vi "CG test stand DAQ main.vi"() -> ()   [LabVIEW 2020]
doc: "This example demonstrates how to read N channels of analog input from a LINX device."
uses:
  <vilib>/MakerHub/LINX/Public/Peripherals/Analog/Analog Read N Chans.vi
  <vilib>/MakerHub/LINX/Private/Local IO/LinxAnalogRead.vi
  <vilib>/MakerHub/LINX/Public/Utilities/Check Channel.vi
  <vilib>/MakerHub/LINX/Public/Utilities/Open Serial.vi
  <vilib>/MakerHub/LINX/Private/Utilties/Generate Error.vi
  <vilib>/Analysis/Matrix/Numeric/Conversions/Array To Matrix - RA.vi
  <vilib>/Utility/file.llb/Write Delimited Spreadsheet (DBL).vi
  <vilib>/MakerHub/LINX/LMH-LINX.lvlib
  <vilib>/Analysis/Matrix/NI_Matrix.lvlib
panel:
  out "Temperatures":dbl[](graph)
  out "Pressures":dbl[](graph)
  out "TC3 (KOhm)":dbl
  out "TC2 (KOhm)":dbl
  out "TC1 (KOhm)":dbl
  out "Throat Pressure (PSI)":dbl
  out "Inlet Pressure (PSI)":dbl
  out "Throat temperature (K)":dbl(slide) scale=0.0..250.0
  out "Inlet temperature (K)":dbl(slide) scale=0.0..250.0
  out "Tank temperature (K)":dbl(slide) scale=0.0..250.0
  out "Throat Pressure (PSI)":dbl(knob) scale=0.0..100.0
  out "Inlet Pressure (PSI)":dbl(knob) scale=0.0..100.0
  out "WRITING TO FILE":bool
  in  "?":bool
  out "error out":errorcluster
  out "Full filepath":string
  in  "Path":path
  in  "File extension":string
  in  "Filename":string
  in  "Wait time (ms)":dbl
  out "Time":timestamp
  in  "Stop Button":bool
  out "Loop Rate (Hz)":u32
  in  "Serial Port":refnum<visa-resource-name>
  # "File I/O"
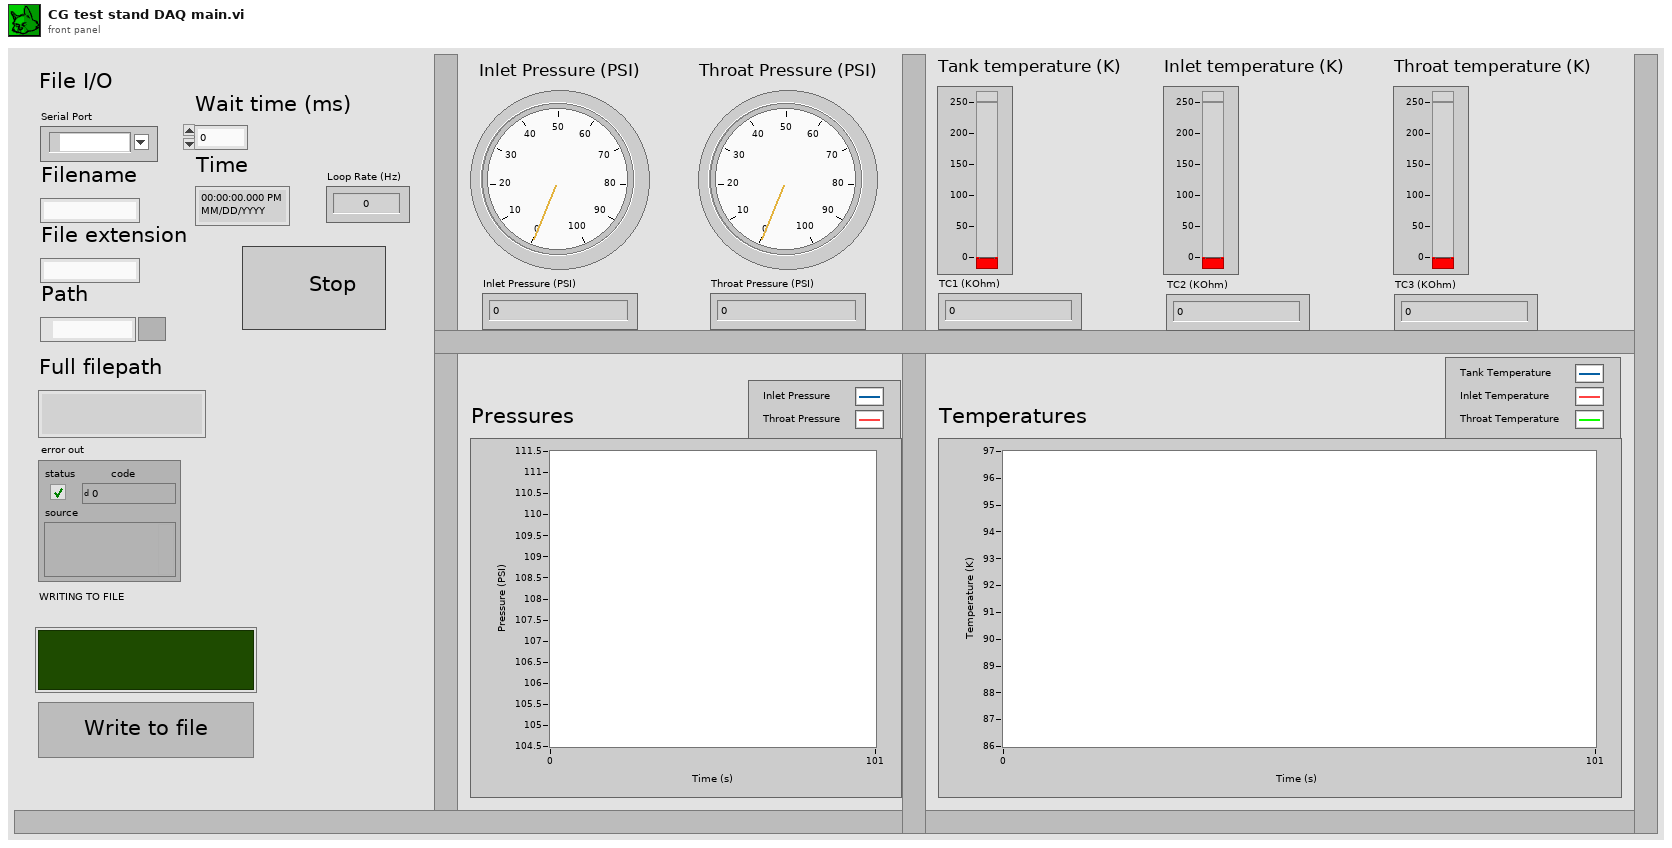
[diagram p1: front panel]
types:
  T1 = typedef "LMH-LINX.lvlib/LINX Ref.ctl" = cluster{"IO":T2, "Interface":T3, "LINX Device Config":T4}
  T2 = typedef "LMH-LINX.lvlib/Platform.ctl" = enum16{"Remote", "Local"}
  T3 = typedef "LMH-LINX.lvlib/Interface.ctl" = enum16{"Serial", "TCP"}
  T4 = typedef "LMH-LINX.lvlib/Device.lvlib/LINX Device Config.ctl" = cluster{"Interface":T3, "COM Port":refnum<visa-resource-name>, "TCP Configuration":T5, "Device Family":u8, "Device ID":u8, "Device Name":string, "TCP Ref":refnum<k5>, "Channels":T6}
  T5 = typedef "LMH-LINX.lvlib/Device.lvlib/TCP Config.ctl" = cluster{"IP Address":string, "Port":u16}
  T6 = typedef "LMH-LINX.lvlib/Channels.ctl" = cluster{"DI":u8[], "DO":u8[], "AI":u8[], "AO":u8[], "PWM":u8[], "QE":u8[], "UART":u8[], "I2C 2":u8[], "SPI":u8[], "CAN":u8[], "Servo":u8[], "AI Ref (V)":dbl, "AI Resolution (Bits)":u8, "AO Ref (V)":dbl, "AO Resolution (Bits)":u8}
  T7 = typedef "NI_Matrix.lvlib/RealMatrix.ctl" = dbl[][]
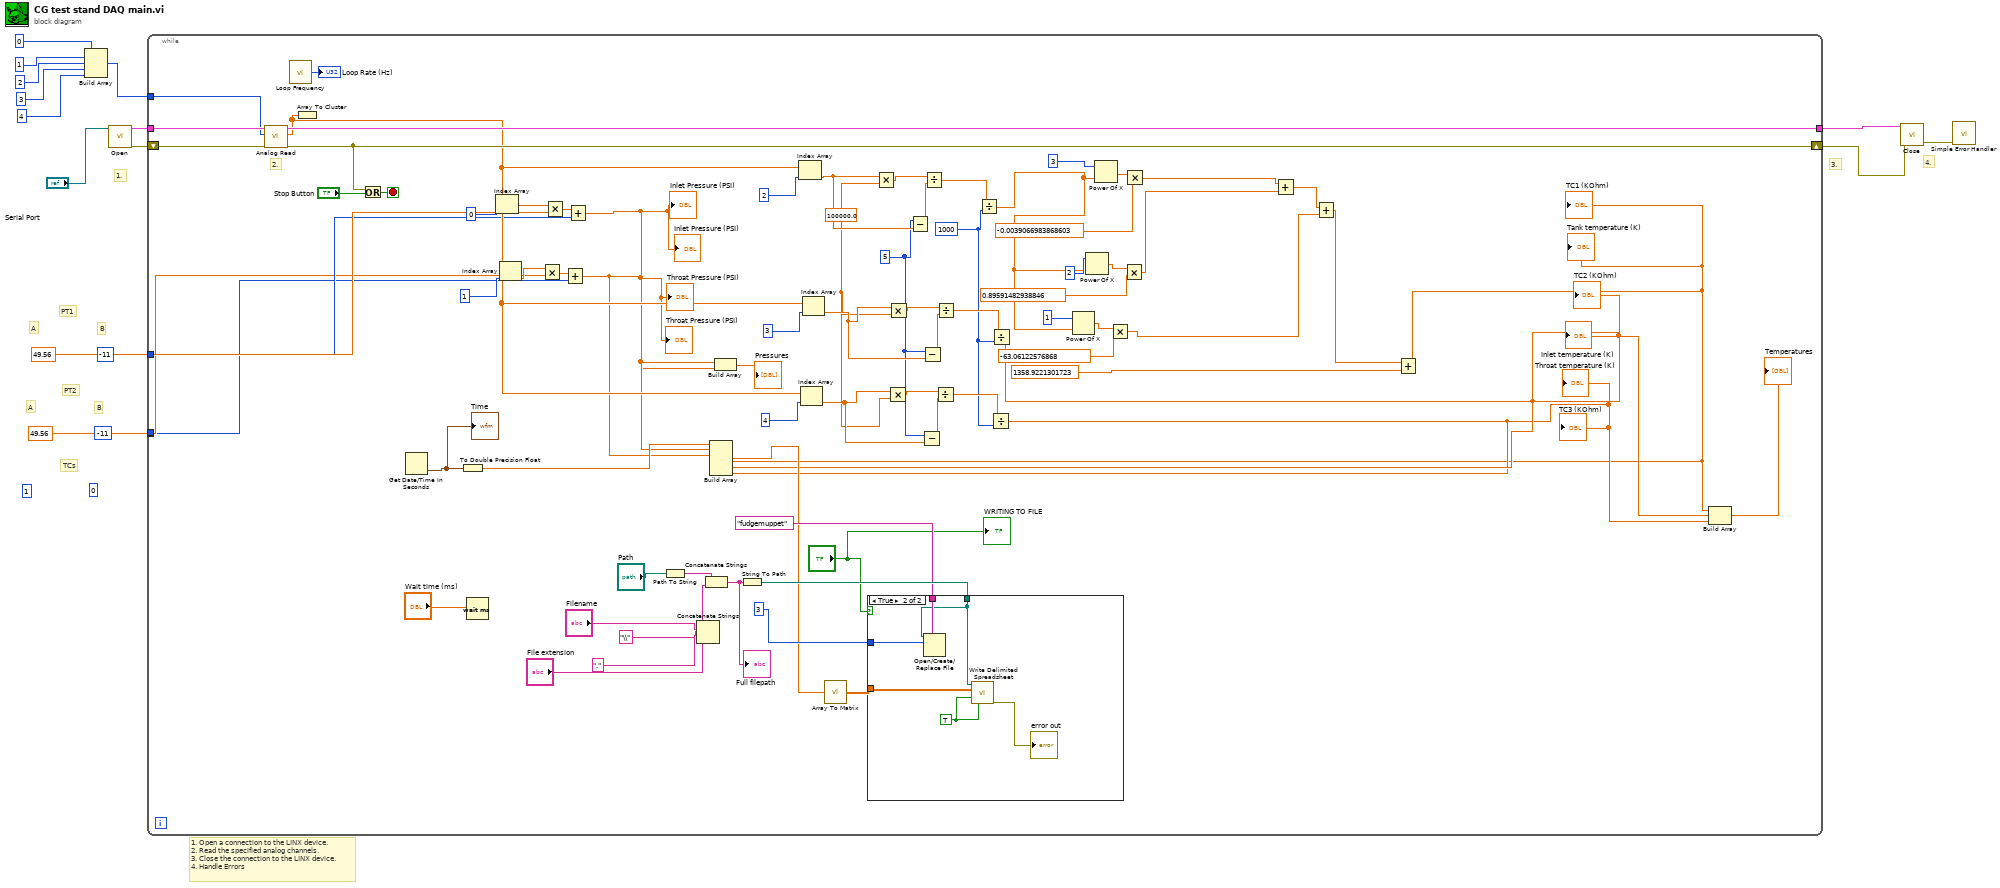
[diagram p0: block diagram]
diagram:
  (unwired) 0
  (unwired) 1
  # "TCs"
  # "B"
  # "A"
  # "PT2"
  # "B"
  # "A"
  # "PT1"
  # "1. Open a connection to the LINX device.\n2. Read the specified analog channels.\n3. Close the connection to the LINX device.\n4. Handle Errors"
  # "4."
  # "3."
  # "1."
  n1 = Build Array(0, 1, 2, 3, 4) -> (w7:i32[])
  n2 = call-poly <vilib>:"Open.vi"("Serial Port"="Serial Port") -> ("Error Out"=w15:errorcluster, "LINX Resource"=w16:T1)  [unwired: 8 in, 1 out]
  n3 = while {
    tunnel: w16 -> [w93]
    tunnel: [w91] -> w14
    shift-right: [w88] -> w13
    shift-left: w15 -> [w92]
    tunnel: w7 -> [w86]
    tunnel: 49.56 -> [w60]
    tunnel: -11 -> [w59]
    tunnel: 49.56 -> [w58]
    tunnel: -11 -> [w57]
    stop <- w90 stop-if-true
    w36 = 1000
    w37 = 5
    w38 = 100000.0
    # "2."
    n4 = call-poly <vilib>:"Analog Read.vi"("Error In"=w92, "AI Channel(s)"=w86, "LINX Resource"=w93) -> ("Error Out"=w88:errorcluster, "Voltages"=w66:dbl[], "LINX Resource"=w91:T1)  [unwired: 5 in, 1 out]
    n5 = call <vilib>:"Loop Frequency.vi"() -> ("Loop Rate (Hz)"=→"Loop Rate (Hz)":u32)
    n6 = Array To Cluster(array=w66) -> ()  [unwired: 1 out]
    n7 = Or(x=w88, y="Stop Button") -> (x .or. y?=w90:bool)
    n8 = Get Date/Time In Seconds() -> (seconds since 1Jan1904=w56:timestamp)
    "Time" <- w56
    n9 = To Double Precision Float(number=w56) -> (double precision float=w55:dbl)
    n10 = Wait (ms)(milliseconds to wait="Wait time (ms)") -> ()  [unwired: 1 out]
    n11 = Index Array(array=w66, index=0) -> (element=w63:dbl)
    n12 = Index Array(array=w66, index=1) -> (element=w64:dbl)
    n13 = Multiply(x=w64, y=w58) -> (x*y=w61:dbl)
    n14 = Multiply(x=w63, y=w60) -> (x*y=w62:dbl)
    n15 = Add(x=w61, y=w57) -> (x+y=w53:dbl)
    "Throat Pressure (PSI)" <- w53
    "Throat Pressure (PSI)" <- w53
    n16 = Add(x=w62, y=w59) -> (x+y=w54:dbl)
    "Inlet Pressure (PSI)" <- w54
    "Inlet Pressure (PSI)" <- w54
    n17 = Path To String(path="Path") -> (string=w82:string)
    n18 = Concatenate Strings("\\", "Filename", ".", "File extension") -> (w81:string)
    n19 = Concatenate Strings(w82, w81) -> (w80:string)
    "Full filepath" <- w80
    n20 = Build Array(w54, w53) -> (→"Pressures":dbl[])
    n21 = String To Path(string=w80) -> (path=w75:path)
    n22 = Index Array(array=w66, index=2) -> (element=w49:dbl)
    n23 = Index Array(array=w66, index=4) -> (element=w39:dbl)
    n24 = Index Array(array=w66, index=3) -> (element=w43:dbl)
    n25 = Multiply(x=w49, y=w38) -> (x*y=w50:dbl)
    n26 = Multiply(x=w39, y=w38) -> (x*y=w42:dbl)
    n27 = Multiply(x=w43, y=w38) -> (x*y=w46:dbl)
    n28 = Subtract(x=w37, y=w49) -> (x-y=w48:dbl)
    n29 = Subtract(x=w37, y=w39) -> (x-y=w41:dbl)
    n30 = Subtract(x=w37, y=w43) -> (x-y=w45:dbl)
    n31 = Divide(x=w50, y=w48) -> (x/y=w47:dbl)
    n32 = Divide(x=w42, y=w41) -> (x/y=w40:dbl)
    n33 = Divide(x=w46, y=w45) -> (x/y=w44:dbl)
    n34 = Divide(x=w47, y=w36) -> (x/y=w17:dbl)
    n35 = Divide(x=w40, y=w36) -> (x/y=w34:dbl)
    "Throat temperature (K)" <- w34
    "TC3 (KOhm)" <- w34
    n36 = Divide(x=w44, y=w36) -> (x/y=w35:dbl)
    "Inlet temperature (K)" <- w35
    "TC2 (KOhm)" <- w35
    n37 = Power Of X(1:w17, 2:1) -> (0:w22:dbl)
    n38 = Power Of X(1:w17, 2:2) -> (0:w23:dbl)
    n39 = Power Of X(1:w17, 2:3) -> (0:w24:dbl)
    n40 = Multiply(x=w22, y=-63.06122576868) -> (x*y=w20:dbl)
    n41 = Multiply(x=w23, y=0.89591482938846) -> (x*y=w21:dbl)
    n42 = Multiply(x=w24, y=-0.0039066983868603) -> (x*y=w18:dbl)
    n43 = Add(x=w18, y=w21) -> (x+y=w19:dbl)
    n44 = Add(x=w19, y=w20) -> (x+y=w26:dbl)
    n45 = Add(x=w26, y=1358.9221301723) -> (x+y=w25:dbl)
    "Tank temperature (K)" <- w25
    "TC1 (KOhm)" <- w25
    n46 = Build Array(w55, w54, w53, w25, w35, w34) -> (w52:dbl[])
    n47 = call-poly <vilib>:"Array To Matrix.vi"("Real 1D Array"=w52) -> ("Real Matrix (Column Vector)"=w51:T7)
    n48 = case shown="True" "?" {
      tunnel: w75 -> [_ w97]
      tunnel: w51 -> [_ w94]
      tunnel: "fudgemuppet" -> [_ w99]
      tunnel: 3 -> [_ w98]
      frame False {
      }
      frame True {
        w95 = TRUE
        n49 = Open/Create/Replace File(file path (use dialog)=w97, prompt=w99, operation (0:open)=w98) -> ()  [unwired: 3 in, 3 out]
        n50 = call-poly <vilib>:"Write Delimited Spreadsheet.vi"("file path (dialog if empty)"=w97, "2D data"=w94, "append to file? (new file:F)"=w95, "transpose? (no:F)"=w95) -> ("error out"=→"error out":errorcluster)  [unwired: 10 in, 1 out]
      }
    }
    n51 = Build Array(w25, w35, w34) -> (→"Temperatures":dbl[])
    "WRITING TO FILE" <- "?"
  }
  n52 = call <vilib>:"Close.vi"("Error In"=w13, "LINX Resource"=w14) -> ("Error Out"=w11:errorcluster)  [unwired: 9 in]
  n53 = call <vilib>:"Simple Error Handler.vi"("error in (no error)"=w11) -> ()  [unwired: 4 in, 5 out]
